vi "Actor Core.vi"(8 "error in":errorcluster, 11 "Microscope in":refnum<class "Microscope.lvclass">) -> (0 "error out":errorcluster, 3 "Actor out":refnum<class "Actor.lvclass">)   [LabVIEW 2020, in "Microscope.lvlib" / "Microscope.lvclass"]
doc: "(<B>Filename</B>: Actor Framework.lvlib:Actor.lvclass:Actor Core.vi)\n\nReceives messages to the actor, reacts to them, and initiates any error handling that may shut the actor down.\n\nDescendant classes may override this VI to append parallel tasks for the actor to complete while it handles messages. Overrides use the Call Parent Class Method node."
uses:
  Microscope.lvclass
  <vilib>/ActorFramework/Actor/Actor.lvclass
  Component/Device/Device/Device.lvclass
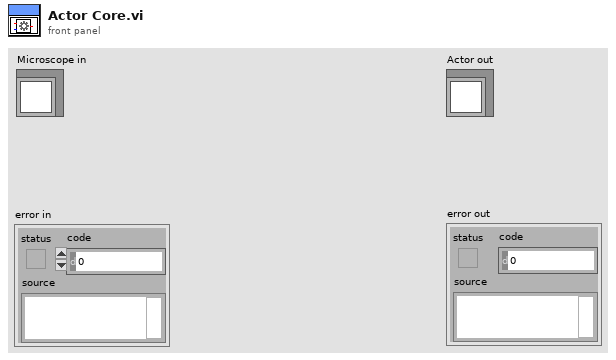
[diagram p1: front panel]
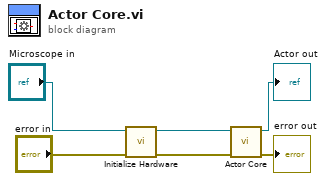
[diagram p0: block diagram]
diagram:
  n1 = call-dynamic "Initialize Hardware.vi"("error in (no error)"="error in", "Microscope in"="Microscope in") -> ("error out"=w3:errorcluster, "Microscope out"=w1:refnum<class "Microscope.lvclass">)  [unwired: 8 in]
  n2 = call-parent "Actor Core.vi"("error in"=w3, "Device in"=w1) -> ("error out"=→"error out":errorcluster, "Actor out"=→"Actor out":refnum<class "Actor.lvclass">)  [unwired: 8 in]
